vi "Status Setpoint 1.vi"(5 "Retry Attempts (0)":i32 min=0, 7 "Unit Address (-1)":i32=-1, 8 "error in (no error)":errorcluster, 11 "VISA resource name (in)":refnum<visa-resource-name>) -> (0 "error out":errorcluster, 2 "Setpoint 1":string, 3 "VISA resource name (out)":refnum<visa-resource-name>)   [LabVIEW 2020, in "Omega Platinum Series.lvlib"]
doc: "Get the setpoint of the controller."
uses:
  <instrlib>/RxnRover/OmegaPlatinumSeriesDriver/Omega Platinum Series.lvlib
panel:
  out "Command":string
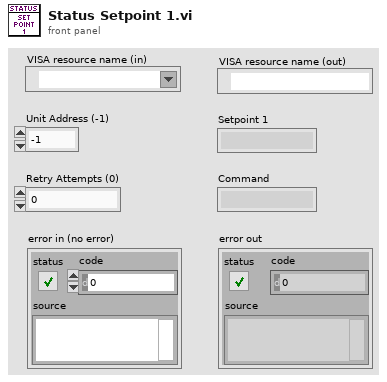
[diagram p1: front panel]
types:
  T1 = typedef "Omega Platinum Series.lvlib/Response.ctl" = cluster{"Unit Address":i32, "Command Class":string, "Command ID":u32, "Parameters":string}
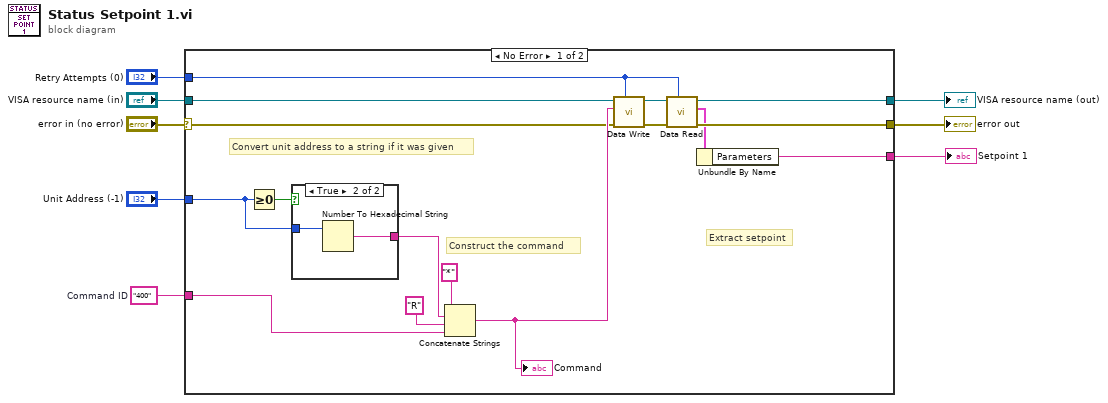
[diagram p0: block diagram]
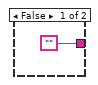
[diagram p2: hidden frame]
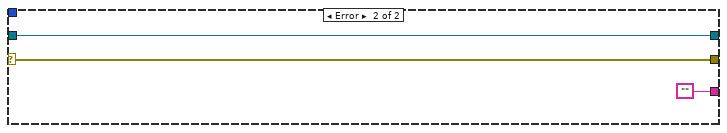
[diagram p3: hidden frame]
diagram:
  w8 = "400"  # Command ID
  n1 = case shown="No Error" "error in (no error)" {
    selector: "error in (no error)" -> [w18 w30]
    tunnel: w8 -> [w12 _]
    tunnel: "Unit Address (-1)" -> [w22 _]
    tunnel: [w14 w30] -> w5
    tunnel: "VISA resource name (in)" -> [w20 w29]
    tunnel: [w15 w29] -> w3
    tunnel: [w10 ""] -> w2
    tunnel: "Retry Attempts (0)" -> [w9 _]
    frame No Error {
      # "Extract setpoint"
      # "Convert unit address to a string if it was given"
      # "Construct the command"
      n2 = Greater Or Equal To 0?(x=w22) -> (x >= 0?=w24:bool)
      n3 = case shown="True" w24 {
        tunnel: w22 -> [_ w27]
        tunnel: ["" w26] -> w21
        frame False {
        }
        frame True {
          n4 = Number To Hexadecimal String(2:w27) -> (0:w26:string)  [unwired: 1 in]
        }
      }
      n5 = Concatenate Strings("*" ("string"), w21, "R" ("string"), w12) -> (w19:string)
      "Command" <- w19
      n6 = call <instrlib>:"Data Write.vi"("Retry Attempts (0)"=w9, "error in (no error)"=w18, "Command"=w19, "VISA Refnum in"=w20) -> ("error out"=w17:errorcluster, "VISA Refnum out"=w16:refnum<visa-resource-name>)  [unwired: 6 in]
      n7 = call <instrlib>:"Data Read.vi"("Retry Attempts (0)"=w9, "error in (no error)"=w17, "VISA Refnum in"=w16) -> ("error out"=w14:errorcluster, "Response Cluster"=w11:T1, "VISA Refnum out"=w15:refnum<visa-resource-name>)  [unwired: 5 in, 1 out]
      n8 = Unbundle By Name(w11) -> ("Parameters"=w10:string)
    }
    frame Error {
    }
  }
  "error out" <- w5
  "VISA resource name (out)" <- w3
  "Setpoint 1" <- w2
